vi "mxwScript_API_XMLTemplateName_AddWireRoutingParameters.vi"(8 "error in (no error)":errorcluster, 10 "routingAlgorithm":T1=enum."AI", 11 "source in":string) -> (0 "error out":errorcluster, 3 "source out":string)   [LabVIEW 2020]
doc: "Add diagram to drop this template into to the template name."
uses:
  codeGenAPISupport.llb/cgAPI_mxwScript_Wire_RoutingAlgorithm.ctl
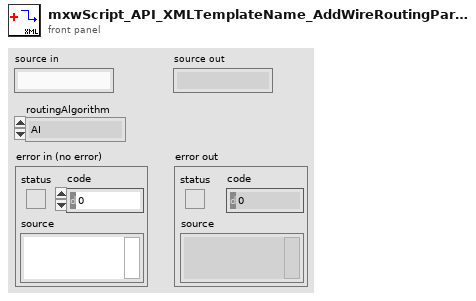
[diagram p1: front panel]
types:
  T1 = typedef "cgAPI_mxwScript_Wire_RoutingAlgorithm.ctl" = enum16{"None", "LV", "AI"}
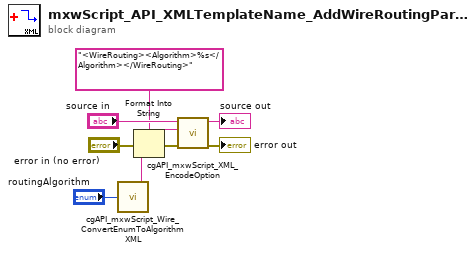
[diagram p0: block diagram]
diagram:
  n1 = call "cgAPI_mxwScript_Wire_ConvertEnumToAlgorithmXML.vi"("routingAlgorithm"="routingAlgorithm") -> ("XML out"=w1:string)  [unwired: 4 out]
  n2 = Format Into String(format string="<WireRouting><Algorithm>%s</Algorithm></WireRouting>" ("control name"), error in="error in (no error)", w1) -> (resulting string=w4:string, error out=w6:errorcluster)  [unwired: 1 in]
  n3 = call "cgAPI_mxwScript_XML_EncodeOption.vi"("error in (no error)"=w6, "otherXML"=w4, "normalTextString"="source in") -> ("error out"=→"error out":errorcluster, "encodedString"=→"source out":string)  [unwired: 7 out]
